vi "graph_cursor.vi"(0 "Colour":i32, 1 "Name":string, 5 "Style":i32, 7 "Point style":i32, 9 "X":dbl, 11 "Y":dbl) -> (4 "Cursor Cluster":T1)   [LabVIEW 2019]
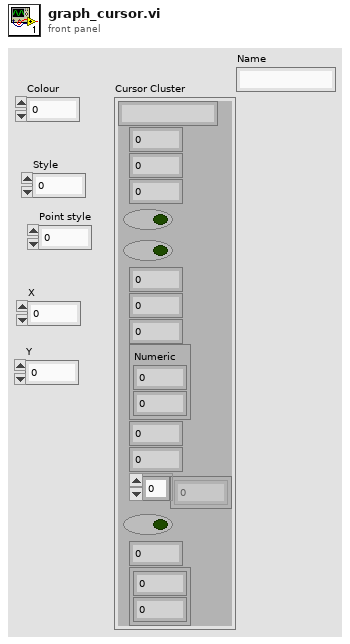
[diagram p1: front panel]
types:
  T1 = cluster{string, i32, i32, i32, bool, bool, i32, i32, i32, cluster{"Numeric":dbl, dbl}, i32, i32, i32[], bool, i32, cluster{dbl, dbl}}
  T2 = cluster{"Name":string, "Colour":i32, "Style":i32, "Point style":i32, bool, bool, i32, i32, i32, cluster{"X":dbl, "Y":dbl}, i32, i32, i32[], bool, i32, cluster{dbl, dbl}}
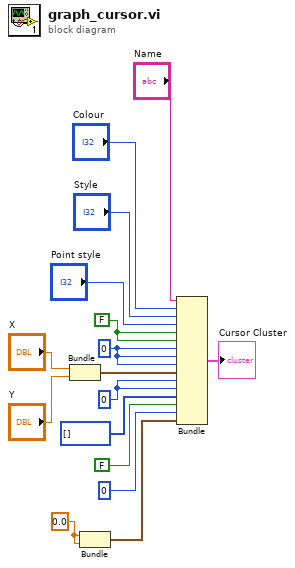
[diagram p0: block diagram]
diagram:
  w13 = 0.0
  w9 = 0
  w7 = 0
  w6 = FALSE
  n1 = Bundle("X"="X", "Y"="Y") -> (w8:cluster{"X":dbl, "Y":dbl})  [unwired: 1 in]
  n2 = Bundle(w13, w13) -> (w14:cluster{dbl, dbl})  [unwired: 1 in]
  n3 = Bundle("Name"="Name", "Colour"="Colour", "Style"="Style", "Point style"="Point style", w6, w6, w7, w7, w7, w8, w9, w9, i32[] [], FALSE, 0, w14) -> (→"Cursor Cluster":T2)  [unwired: 1 in]
